vi "Teleop.vi"(10 "Match Info":T1={"Autonomous Elapsed Seconds"=0.0, "TeleOp Elapsed Seconds"=0.0, "Disabled Elapsed Seconds"=0.0, "Visited Autonomous"=FALSE, "Visited TeleOp"=FALSE, "Visited Disabled"=FALSE, "Autonomous Settings"={"Autonomous Style"=enum."Independent", "VI Refnum"=refnum}}, 11 "Call Context":T2) -> ()   [LabVIEW 2016]
doc: "This VI is called for each TeleOp packet received from the DS where the robot is not disabled. It is often used to read from the joysticks and update I/O or to update setpoints for timed control loops. It should complete and return within 20 milliseconds or it may miss DS packets."
uses:
  <vilib>/Rock Robotics/WPI/DriverStation/WPI_DriverStationDerivedRobotMode.ctl
  <vilib>/Rock Robotics/WPI/DriverStation/WPI_DriverStationMatch Info.ctl
  <vilib>/Rock Robotics/WPI/Solenoid/WPI_SolenoidValue.ctl
  <vilib>/Rock Robotics/WPI/ThirdParty/CanMotor/TalonSRX/WPI_CANTalonSRX_APIControlMode.ctl
  <vilib>/Rock Robotics/WPI/Utilities/WPI_GetSetVariantRefNum.vi
  Robot Global Data.vi
  <vilib>/Rock Robotics/WPI/Solenoid/WPI_SolenoidSetEnum.vi
panel:
  in  "F":dbl
  in  "P":dbl
  in  "Numeric":dbl=220.0 format="%#_13g"
  out "Right Current":dbl
  out "Left Current":dbl
  out "Right Encoder":dbl
  out "Left Encoder":dbl
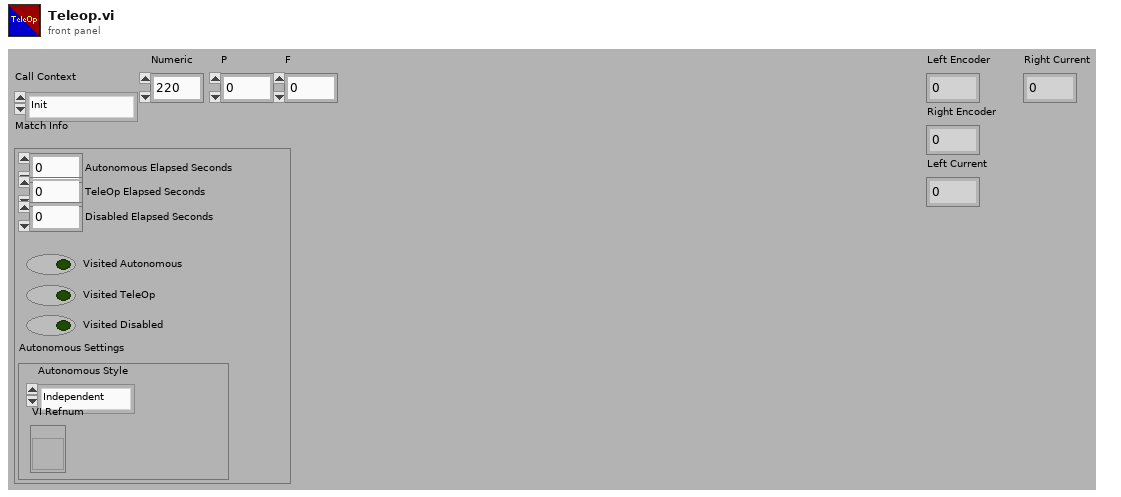
[diagram p1: front panel]
types:
  T1 = typedef "WPI_DriverStationMatch Info.ctl" = cluster{"Autonomous Elapsed Seconds":dbl, "TeleOp Elapsed Seconds":dbl, "Disabled Elapsed Seconds":dbl, "Visited Autonomous":bool, "Visited TeleOp":bool, "Visited Disabled":bool, "Autonomous Settings":cluster{"Autonomous Style":enum16{"Iterative", "Independent"}, "VI Refnum":refnum<vi>}}
  T2 = typedef "WPI_DriverStationDerivedRobotMode.ctl" = enum16{"Init", "Execute", "Stop"}
  T3 = typedef "WPI_SolenoidValue.ctl" = enum16{"Off", "On", "Forward", "Reverse"}
  T4 = typedef "WPI_JoystickDevRef.ctl" = cluster{"Device":T5}
  T5 = typedef "WPI_JoystickDeviceEnum.ctl" = enum16{"USB 0", "USB 1", "USB 2", "USB 3", "USB 4", "USB 5"}
  T6 = typedef "WPI_SolenoidDevRef.ctl" = cluster{"DevStatus":errorcluster, "Pneumatics Control Module":u8, "Forward Solenoid Channel":T7, "Reverse Solenoid Channel":T7}
  T7 = typedef "WPI_SolenoidChannel.ctl" = enum8{"Solenoid 0", "Solenoid 1", "Solenoid 2", "Solenoid 3", "Solenoid 4", "Solenoid 5", "Solenoid 6", "Solenoid 7", "Invalid"}
  T8 = typedef "WPI_MotorControlDeviceRef.ctl" = cluster{"DeviceStatus":errorcluster, "Type":T9, "PWM":cluster{"PWM Channel":T10, "DeadBand":T11}, "CAN":cluster{"Device Number":u8, "SetOutput VI Ref":variant, "GetOutput VI Ref":variant, "Enable VI Ref":variant, "Disable VI Ref":variant, "Data":variant}, "Invert":bool}
  T9 = typedef "WPI_MotorControlType.ctl" = enum16{"PWM", "CAN"}
  T10 = typedef "FPGA_DIOPWMChannel.ctl" = enum8{"PWM 0", "PWM 1", "PWM 2", "PWM 3", "PWM 4", "PWM 5", "PWM 6", "PWM 7", "PWM 8", "PWM 9", "PWM MXP 0", "PWM MXP 1", "PWM MXP 2", "PWM MXP 3", "PWM MXP 4", "PWM MXP 5", "PWM MXP 6", "PWM MXP 7", "PWM MXP 8", "PWM MXP 9", "Invalid"}
  T11 = typedef "WPI_PWMDeadband.ctl" = cluster{"Name":string, "maxPositivePwm":i32, "minPositivePwm":i32, "centerPwm":i32, "maxNegativePwm":i32, "minNegativePwm":i32, "angularRange":u16}
  T12 = typedef "WPI_CANTalonSRX_GlobalStatus.ctl" = cluster{"Applied Throttle":dbl, "Module Enabled":bool, "CAN Error":errorcluster, "Closed Loop Error":dbl, "Forward Limit Switch Closed":bool, "Reverse Limit Switch Closed":bool, "Sensor Position":dbl, "Sensor Velocity":dbl, "Current":dbl, "Sticky Fault - Over Temp":bool, "Sticky Fault - Under Voltage":bool, "Sticky Fault - Forward Limit":bool, "Sticky Fault - Reverse Limit":bool, "Sticky Fault - Forward Soft Limit":bool, "Sticky Fault - Reverse Soft Limit":bool, "Brake is Enabled":bool, "Encoder Position":dbl, "Encoder Velocity":dbl, "Encoder Index Count":dbl, "Encoder A Pin State":bool, "Encoder B Pin State":bool, "Encoder Index Pin State":bool, "Analog In":dbl, "Analog In Velocity":dbl, "Temperature (C)":dbl, "Battery Voltage":dbl, "Control 5 Is Supported":bool, "Current Profile Slot Select":dbl, "Pos Div 8":bool, "Vel Div 4":bool, "Pulse Width Position":i32, "Pulse Width Velocity":i32, "Pulse Width Rise To Rise (us)":i32, "Pulse Width Rise To Fall (us)":i32, "Mot Prof Active Is Under Run":bool, "Mot Prof Active Has Under Run":bool, "Mot Prof Active Is Last":bool, "Mot Prof Active Velocity Only":bool, "Mot Prof Active Is Valid":bool, "Mot Prof Buffer Is Full":bool, "Mot Prof Active Profile Slot Select":i32, "Mot Prof NextID":i32, "Mot Prof Count":i32, "Mot Prof Active Velocity":dbl, "Mot Prof Active Position":dbl, "Mot Prof Output Enable":i32}
  T13 = typedef "WPI_CANTalonSRX_APIControlMode.ctl" = enum8{"Percent VBus", "Speed", "Position", "Slave", "Unchanged / Invalid", "Voltage Compensation", "Current", "Motion Profile", "Motion Magic"}
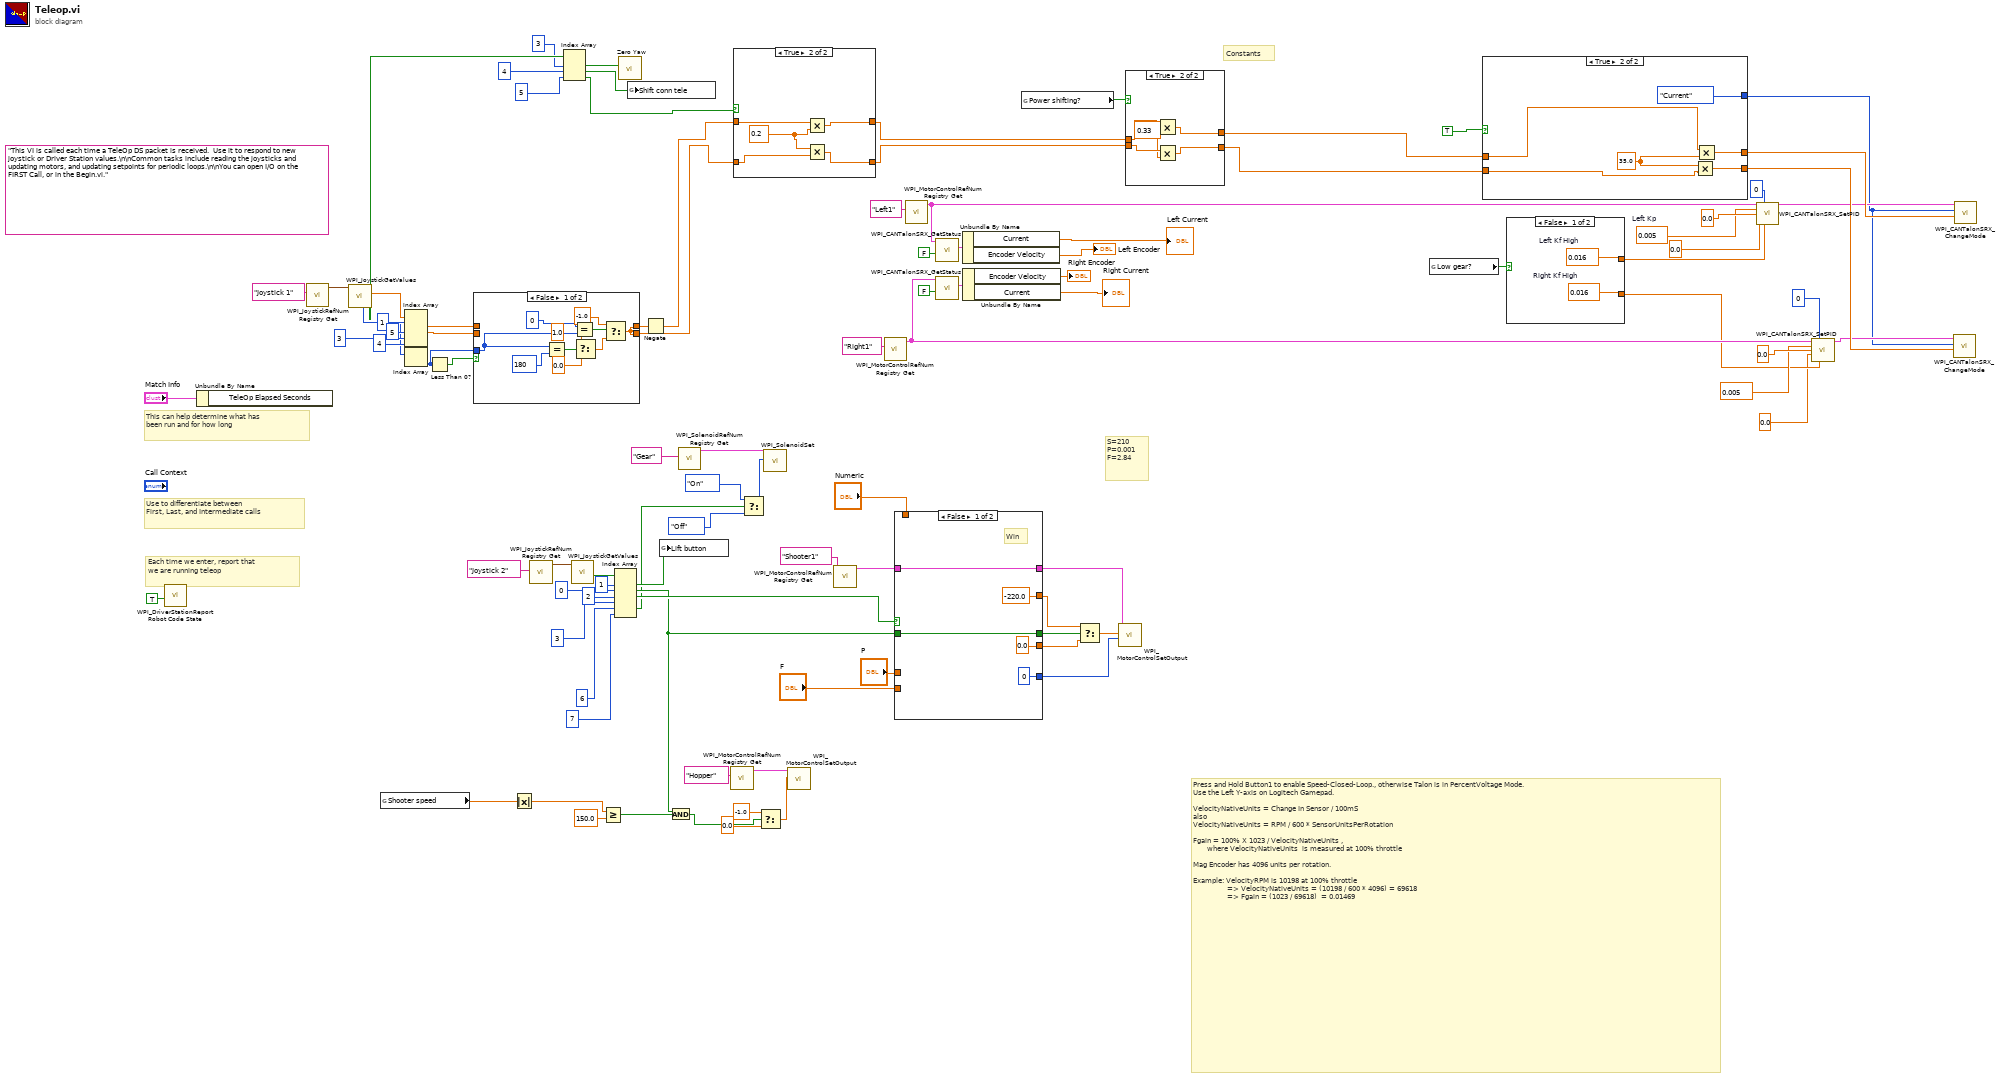
[diagram p0: block diagram]
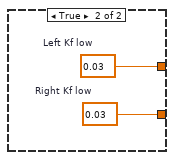
[diagram p3: hidden frame]
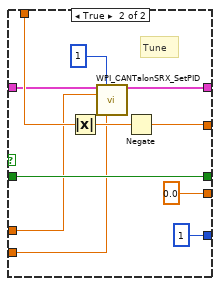
[diagram p5: hidden frame]
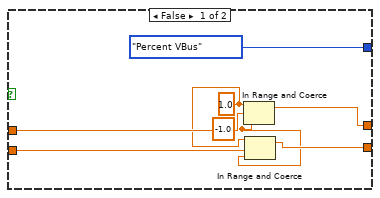
[diagram p6: hidden frame]
diagram:
  w24 = 0.005  # Left Kp
  (unwired) "This VI is called each time a TeleOp DS packet is received.  Use it to respond to new joystick or Driver Station values.\n\nCommon tasks include reading the joysticks and updating motors, and updating setpoints for periodic loops.\n\nYou can open I/O on the FIRST Call, or in the Begin.vi."
  # "S=210\nP=0.001\nF=2.84"
  # "Constants"
  # "Press and Hold Button1 to enable Speed-Closed-Loop., otherwise Talon is in PercentVoltage Mode.  \nUse the Left Y-axis on Logitech Gamepad.\n\nVelocityNativeUnits = Change In Sensor / 100mS\nalso\nVelocityNativeUnits = RPM / 600 * SensorUnitsPerRotation\n\nFgain = 100% X 1023 / VelocityNativeUnits , \n       where VelocityNativeUnits  is measured at 100% throttle\n\nMag Encoder has 4096 units per rotation.\n\nExample: VelocityRPM is 10198 at 100% throttle\n                 => VelocityNativeUnits = (10198 / 600 * 4096) = 69618\n                 => Fgain = (1023 / 69618)  = 0.01469"
  # "Each time we enter, report that\nwe are running teleop"
  # "Use to differentiate between\nFirst, Last, and Intermediate calls"
  # "This can help determine what has\nbeen run and for how long"
  n1 = call <vilib>:"WPI_DriverStationReport Robot Code State.vi"("TeleOp"=TRUE ("Autonomous")) -> ()  [unwired: 10 in, 1 out]
  n2 = Unbundle By Name("Match Info") -> ()  [unwired: 1 out]
  n3 = call <vilib>:"WPI_JoystickRefNum Registry Get.vi"("refnum name"="Joystick 1") -> ("JoystickDevRef"=w92:T4)  [unwired: 9 in, 1 out]
  n4 = call <vilib>:"WPI_JoystickGetValues.vi"("JoystickDevRef"=w92) -> ("Buttons"=w28:bool[], "Axes"=w91:dbl[], "POVs"=w37:i16[])  [unwired: 6 in, 2 out]
  n5 = global read "Robot Global Data.vi" "Shooter speed"() -> (w76:dbl)
  n6 = Index Array(array=w91, index #1=1 ("index"), index #2=5 ("index"), index #3=3 ("index"), index #4=4 ("index")) -> (element #1=w31:dbl, element #2=w30:dbl)  [unwired: 2 out]
  n7 = Index Array(array=w37) -> (element=w29:i16)  [unwired: 1 in]
  n8 = Less Than 0?(x=w29) -> (x < 0?=w33:bool)
  n9 = case shown="False" w33 {
    tunnel: [w107 w109] -> w32
    tunnel: w31 -> [_ w109]
    tunnel: [w107 w108] -> w6
    tunnel: w30 -> [_ w108]
    tunnel: w29 -> [w104 _]
    frame False {
      n10 = Equal?(x=w104, y=i16 180) -> (x = y?=w105:bool)
      n11 = Equal?(x=i16 0, y=w104) -> (x = y?=w100:bool)
      n12 = Select(t=1.0, s=w105, f=0.0) -> (s? t:f=w106:dbl)
      n13 = Select(t=-1.0, s=w100, f=w106) -> (s? t:f=w107:dbl)
    }
    frame True {
    }
  }
  n14 = Absolute Value(x=w76) -> (abs(x)=w65:dbl)
  n15 = call <vilib>:"WPI_JoystickRefNum Registry Get.vi"("refnum name"="Joystick 2") -> ("JoystickDevRef"=w80:T4)  [unwired: 9 in, 1 out]
  n16 = Index Array(array=w28, index #1=3 ("index"), index #2=4 ("index"), index #3=5 ("index")) -> (element #1=w27:bool, element #2=w1:bool, element #3=w2:bool)
  n17 = call <vilib>:"WPI_JoystickGetValues.vi"("JoystickDevRef"=w80) -> ("Buttons"=w79:bool[])  [unwired: 6 in, 4 out]
  n18 = Greater Or Equal?(x=w65, y=150.0) -> (x >= y?=w44:bool)
  n19 = Index Array(array=w79, index #1=1 ("index"), index #2=0 ("index"), index #3=2 ("index"), index #4=3 ("index"), index #5=6, index #6=7) -> (element #1=w78:bool, element #2=w69:bool, element #3=w71:bool, element #5=w8:bool)  [unwired: 2 out]
  n20 = call <vilib>:"Zero Yaw.vi"("Zero"=w27) -> ()  [unwired: 11 in]
  n21 = global write "Robot Global Data.vi" "Shift conn tele"(w1) -> ()
  n22 = Negate(x=w32) -> (-x=w7:dbl)
  n23 = global write "Robot Global Data.vi" "Lift button"(w78) -> ()
  n24 = And(x=w69, y=w44) -> (x .and. y?=w36:bool)
  n25 = call <vilib>:"WPI_SolenoidRefNum Registry Get.vi"("refnum name"="Gear") -> ("SolenoidDevRef"=w13:T6)  [unwired: 9 in, 1 out]
  n26 = call <vilib>:"WPI_MotorControlRefNum Registry Get.vi"("refnum name"="Hopper") -> ("MotorControlDevRef"=w85:T8)  [unwired: 9 in, 1 out]
  n27 = case shown="True" w2 {
    tunnel: w7 -> [w110 w116]
    tunnel: w6 -> [w111 w114]
    tunnel: [w111 w113] -> w4
    tunnel: [w110 w112] -> w5
    frame False {
    }
    frame True {
      w115 = 0.2
      n28 = Multiply(x=w116, y=w115) -> (x*y=w112:dbl)
      n29 = Multiply(x=w115, y=w114) -> (x*y=w113:dbl)
    }
  }
  n30 = Select(t=WPI_SolenoidValue."On" ("Value"), s=w8, f=WPI_SolenoidValue."Off" ("Value")) -> (s? t:f=w9:T3)
  n31 = Select(t=-1.0, s=w36, f=0.0) -> (s? t:f=w83:dbl)
  n32 = call-poly <vilib>:"WPI_SolenoidSet.vi"("Value"=w9, "SolenoidDevRef"=w13) -> ()  [unwired: 8 in, 2 out]
  n33 = call <vilib>:"WPI_MotorControlSetOutput.vi"("Output"=w83, "MotorControlDevRef"=w85) -> ()  [unwired: 7 in, 3 out]
  n34 = call <vilib>:"WPI_MotorControlRefNum Registry Get.vi"("refnum name"="Shooter1") -> ("MotorControlDevRef"=w61:T8)  [unwired: 9 in, 1 out]
  n35 = call <vilib>:"WPI_MotorControlRefNum Registry Get.vi"("refnum name"="Right1") -> ("MotorControlDevRef"=w52:T8)  [unwired: 9 in, 1 out]
  n36 = case shown="False" w71 {
    tunnel: [0.0 ("f") 0.0] -> w87
    tunnel: [-220.0 ("Numeric") w128] -> w67
    tunnel: [w120 w132] -> w70
    tunnel: w69 -> [w120 w132]
    tunnel: "Numeric" -> [_ w130]
    tunnel: [w117 w125] -> w46
    tunnel: w61 -> [w117 w126]
    tunnel: "P" -> [_ w123]
    tunnel: "F" -> [_ w122]
    tunnel: [u8 0 ("options") u8 1 ("options")] -> w45
    frame False {
      # "Win"
    }
    frame True {
      # "Tune"
      n37 = Absolute Value(x=w130) -> (abs(x)=w129:dbl)
      n38 = call <vilib>:"WPI_CANTalonSRX_SetPID.vi"("CAN Talon SRX Ref"=w126, "Parameter Slot"=u8 1, "P"=w123, "F"=w122) -> ("CAN Talon SRX Ref"=w125:T8)  [unwired: 10 in, 1 out]
      n39 = Negate(x=w129) -> (-x=w128:dbl)
    }
  }
  n40 = call <vilib>:"WPI_MotorControlRefNum Registry Get.vi"("refnum name"="Left1") -> ("MotorControlDevRef"=w53:T8)  [unwired: 9 in, 1 out]
  n41 = call <vilib>:"WPI_CANTalonSRX_GetStatus.vi"("Clear Sticky Faults"=FALSE, "CAN Talon SRX Ref"=w53) -> ("Talon SRX Status"=w54:T12)  [unwired: 7 in, 2 out]
  n42 = call <vilib>:"WPI_CANTalonSRX_GetStatus.vi"("Clear Sticky Faults"=FALSE, "CAN Talon SRX Ref"=w52) -> ("Talon SRX Status"=w56:T12)  [unwired: 7 in, 2 out]
  n43 = Unbundle By Name(w54) -> ("Current"=→"Left Current":dbl, "Encoder Velocity"=→"Left Encoder":dbl)
  n44 = Unbundle By Name(w56) -> ("Encoder Velocity"=→"Right Encoder":dbl, "Current"=→"Right Current":dbl)
  n45 = global read "Robot Global Data.vi" "Power shifting?"() -> (w38:bool)
  n46 = Select(t=w67, s=w70, f=w87) -> (s? t:f=w47:dbl)
  n47 = call <vilib>:"WPI_MotorControlSetOutput.vi"("options"=w45, "Output"=w47, "MotorControlDevRef"=w46) -> ()  [unwired: 6 in, 3 out]
  n48 = case shown="True" w38 {
    tunnel: w5 -> [w134 w139]
    tunnel: [w134 w137] -> w41
    tunnel: w4 -> [w133 w138]
    tunnel: [w133 w136] -> w40
    frame False {
    }
    frame True {
      w135 = 0.33
      n49 = Multiply(x=w139, y=w135) -> (x*y=w137:dbl)
      n50 = Multiply(x=w138, y=w135) -> (x*y=w136:dbl)
    }
  }
  n51 = global read "Robot Global Data.vi" "Low gear?"() -> (w14:bool)
  n52 = case shown="True" TRUE {
    tunnel: [WPI_CANTalonSRX_APIControlMode."Percent VBus" ("Control Mode") WPI_CANTalonSRX_APIControlMode."Current" ("Control Mode")] -> w17
    tunnel: [w142 w151] -> w90
    tunnel: [w143 w147] -> w89
    tunnel: w41 -> [w145 w150]
    tunnel: w40 -> [w144 w149]
    frame False {
      w141 = -1.0 ("lower limit")
      w140 = 1.0 ("upper limit")
      n53 = In Range and Coerce(upper limit=w140, x=w145, lower limit=w141) -> (coerced(x)=w142:dbl)  [unwired: 1 out]
      n54 = In Range and Coerce(upper limit=w140, x=w144, lower limit=w141) -> (coerced(x)=w143:dbl)  [unwired: 1 out]
    }
    frame True {
      w148 = 35.0
      n55 = Multiply(x=w148, y=w149) -> (x*y=w147:dbl)
      n56 = Multiply(x=w150, y=w148) -> (x*y=w151:dbl)
    }
  }
  n57 = case shown="False" w14 {
    tunnel: [w154 w156] -> w23
    tunnel: [w153 w155] -> w21
    frame False {
      w153 = 0.016  # Right Kf High
      w154 = 0.016  # Left Kf High
    }
    frame True {
      w155 = 0.03  # Right Kf low
      w156 = 0.03  # Left Kf low
    }
  }
  n58 = call <vilib>:"WPI_CANTalonSRX_SetPID.vi"("CAN Talon SRX Ref"=w53, "Parameter Slot"=u8 0, "P"=w24, "I"=0.0, "D"=0.0 ("Kd left"), "F"=w23) -> ("CAN Talon SRX Ref"=w64:T8)  [unwired: 8 in, 1 out]
  n59 = call <vilib>:"WPI_CANTalonSRX_SetPID.vi"("CAN Talon SRX Ref"=w52, "Parameter Slot"=u8 0, "P"=0.005 ("Right Kp"), "I"=0.0, "D"=0.0 ("Kd Right"), "F"=w21) -> ("CAN Talon SRX Ref"=w59:T8)  [unwired: 8 in, 1 out]
  n60 = call <vilib>:"WPI_CANTalonSRX_ChangeMode.vi"("Output"=w89, "Control Mode"=w17, "CAN Talon SRX Ref"=w59) -> ()  [unwired: 7 in, 2 out]
  n61 = call <vilib>:"WPI_CANTalonSRX_ChangeMode.vi"("Output"=w90, "Control Mode"=w17, "CAN Talon SRX Ref"=w64) -> ()  [unwired: 7 in, 2 out]
